vi "test frame felica ask.vi"() -> ()   [LabVIEW 2019]
uses:
  <vilib>/Analysis/3filter.llb/Filter Passband Type.ctl
  <vilib>/addons/Modulation/Analog/support/mod_Set Error Source.vi
  <vilib>/addons/Modulation/Digital/Support/Common/Validators/mod_Generate Filter Coefficients Validate.vi
  <vilib>/addons/Modulation/Digital/General/subVIs/mod_Generate Filter Coefficients.vi
  <vilib>/addons/Modulation/Digital/General/MT Generate ASK system parameters (M).vi
  <vilib>/Waveform/DWDTOps.llb/DWDT Binary U8 to Digital.vi
  <vilib>/addons/Modulation/Analog/MT Modulate AM (DSB).vi
  <vilib>/addons/Modulation/Analog/MT Upconvert Baseband (Real).vi
  <vilib>/express/express analysis/Spectral/Block/exnSpectralBlock spectral measurements RMS poly.vi
  <vilib>/express/express analysis/Spectral/Block/exnSpectralBlock spectral measurements RMS WFM.vi
  <vilib>/Analysis/3filter.llb/Butterworth Filter (DBL).vi
  <vilib>/express/express analysis/Spectral/XNode/ExpressSpectralMeasurementsBlockNode.xnode
  <vilib>/addons/Modulation/niDMT.lvlib
  <vilib>/addons/Modulation/niAMT.lvlib
  <vilib>/Analysis/NI_AALBase.lvlib
panel:
  out "video signal 3":cluster{"t0":dbl, "dt":dbl, "Y":dbl[]}(graph)
  out "video signal 2":cluster{"t0":dbl, "dt":dbl, "Y":dbl[]}(graph)
  in  "command":enum16{"WUP_REQ"}(ring)
  out "error":i32
  out "spectrum analog signal 3":cluster{"t0":dbl, "dt":dbl, "Y":dbl[]}(graph)
  out "Analog signal 2":waveform(dbl)(graph)
  out "spectrum analog signal 2":cluster{"t0":dbl, "dt":dbl, "Y":dbl[]}(graph)
  out "spectrum analog signal":cluster{"t0":dbl, "dt":dbl, "Y":dbl[]}(graph)
  in  "CARRIER (hz)":dbl
  in  "BIT RATE":dbl
  out "LENGHT":u8[](array[numeric]) format="%x"
  out "dt":dbl
  out "Analog signal":waveform(dbl)(graph)
  out "video signal":cluster{"t0":dbl, "dt":dbl, "Y":dbl[]}(graph)
  out "Digital SIGNAL":digitalwaveform(graph)
  out "CRC":u8[](array[numeric]) format="%x"
  in  "Data":u8[](array[numeric]) format="%x"
  in  "SYNC":u8[](array[numeric]) format="%x"
  in  "Preambula":u8[](array[numeric]) format="%x"
  # "0"
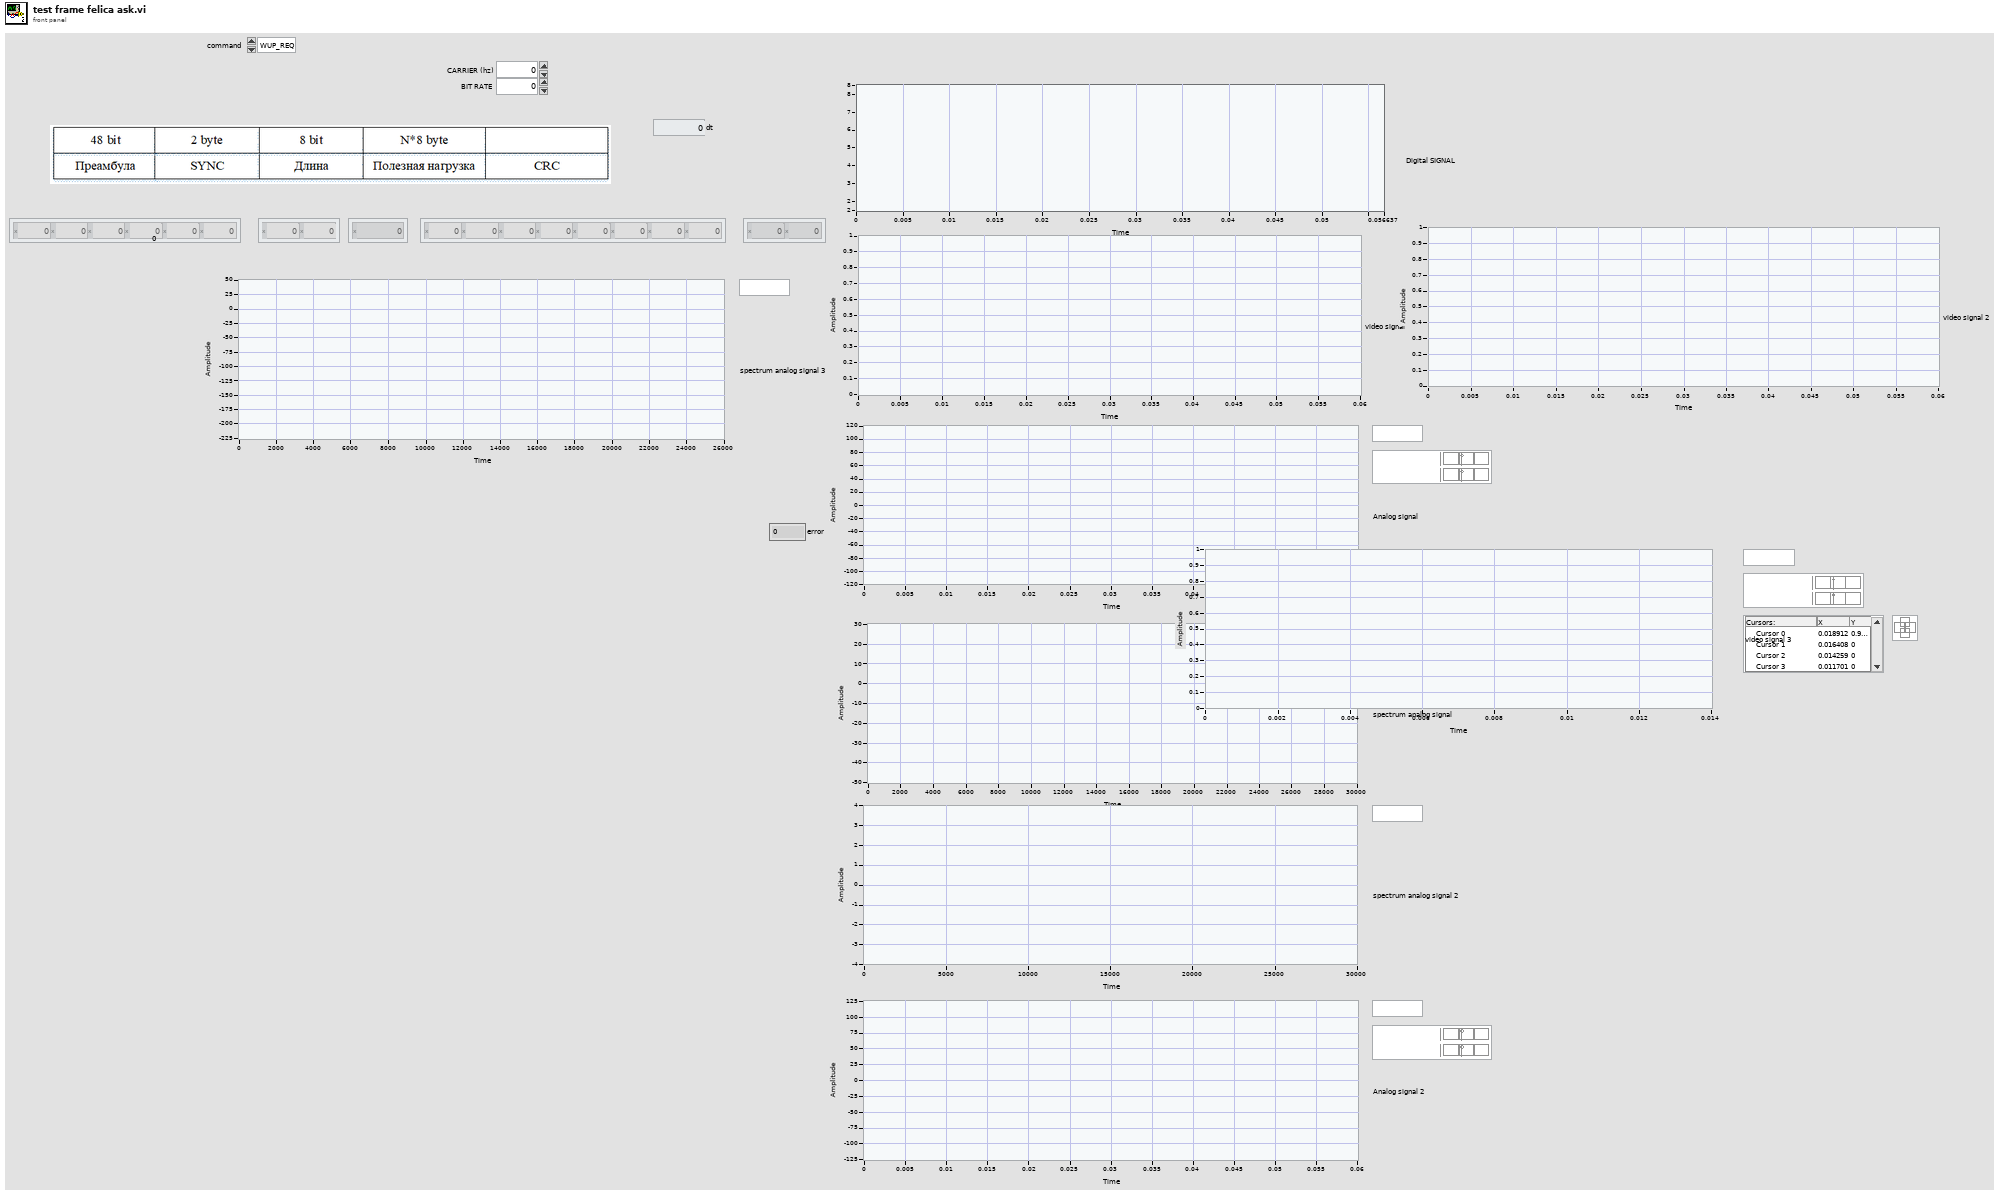
[diagram p1: front panel]
types:
  T1 = enum16{"none", "Raised Cosine", "Root Raised Cos", "Gaussian"}
  T2 = enum16{"FSK", "PSK", "QAM", "MSK", "PAM", "ASK", "CPM"}
  T3 = typedef "NI_AALBase.lvlib/Filter Passband Type.ctl" = enum32{"Lowpass", "Highpass", "Bandpass", "Bandstop"}
  T4 = cluster{"samples per symbol (16)":i32, "symbol map":cdb[]}
  T5 = typedef "niAMT.lvlib/Complex Data Waveform.ctl" = cluster{"t0":dbl, "dt":dbl, "Y":cdb[]}
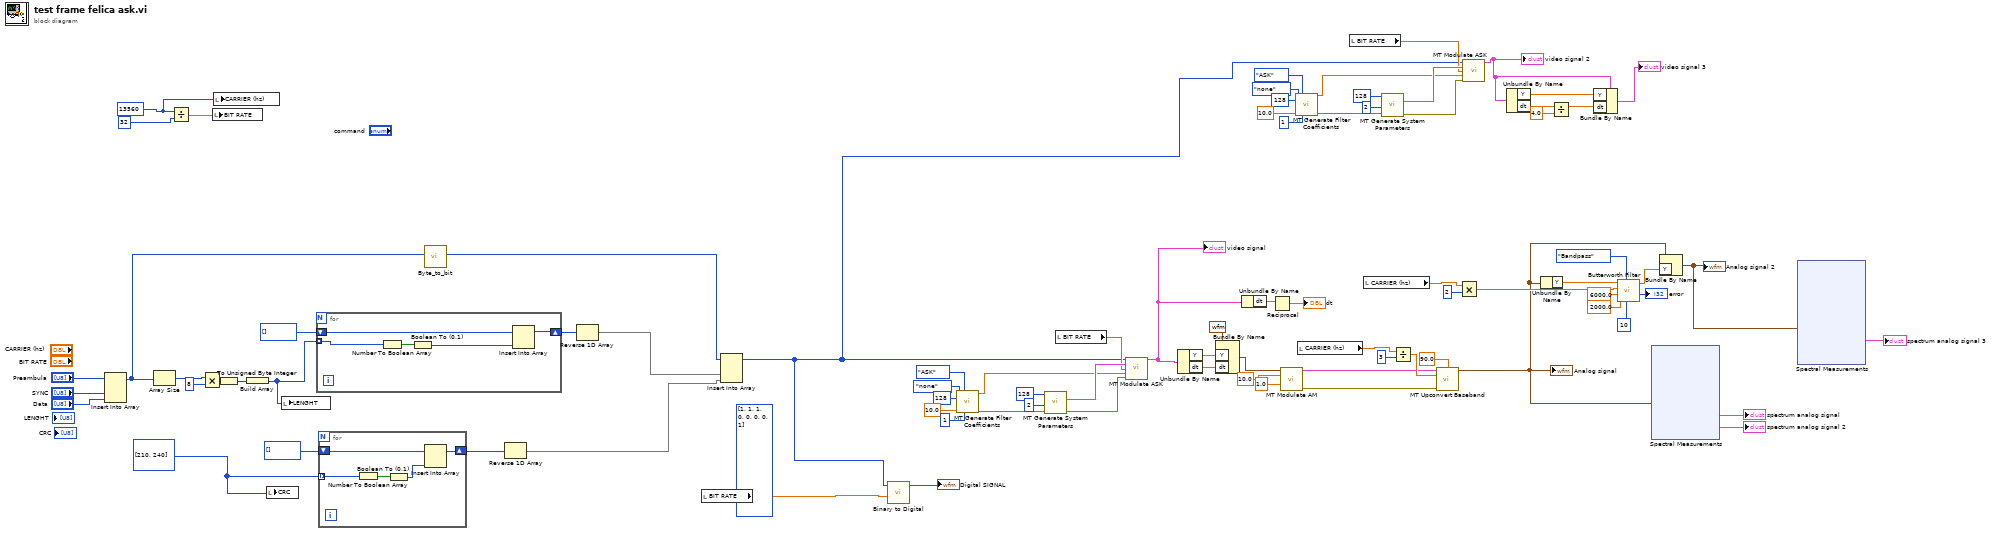
[diagram p0: block diagram]
diagram:
  (unwired) i16[] [1, 1, 1, 0, 0, 0, 0, 1] ("output array")
  w14 = 128 ("pulse shaping samples per symbol (16)")
  w45 = u32 13560
  w61 = 128 ("pulse shaping samples per symbol (16)")
  w48 = u8[] [210, 240] ("CRC")
  n1 = Insert Into Array(array="Preambula", new element #1="SYNC", new element #2="Data") -> (w79:u8[])  [unwired: 1 in]
  n2 = Array Size(array=w79) -> (size(s)=w78:i32)
  n3 = Divide(x=w45, y=u32 32) -> (x/y=w50:dbl)
  n4 = Multiply(x=w78, y=8) -> (x*y=w76:i32)
  n5 = local write "BIT RATE"(w50) -> ()
  n6 = local write "CARRIER (hz)"(w45) -> ()
  n7 = To Unsigned Byte Integer(number=w76) -> (unsigned 8bit integer=w75:u8)
  n8 = Build Array(w75) -> (w47:u8[])
  n9 = local write "CRC"(w48) -> ()
  n10 = local write "LENGHT"(w47) -> ()
  n11 = for {
    tunnel: w47 -> [w87] mode=indexing
    shift-right: [w85] -> w72
    shift-left: i16[] [] -> [w84]
    n12 = Number To Boolean Array(number=w87) -> (Boolean array=w88:bool[])
    n13 = Boolean To (0,1)(Boolean=w88) -> (0, 1=w86:i16[])
    n14 = Insert Into Array(array=w84, new element=w86) -> (w85:i16[])  [unwired: 1 in]
  }
  n15 = for {
    tunnel: w48 -> [w90] mode=indexing
    shift-right: [w92] -> w73
    shift-left: i16[] [] -> [w89]
    n16 = Number To Boolean Array(number=w90) -> (Boolean array=w93:bool[])
    n17 = Boolean To (0,1)(Boolean=w93) -> (0, 1=w91:i16[])
    n18 = Insert Into Array(array=w89, new element=w91) -> (w92:i16[])  [unwired: 1 in]
  }
  n19 = call "Byte_to_bit.vi"("Array of byte"=w79) -> ("Arrray of bit"=w70:u8[])  [unwired: 6 in, 2 out]
  n20 = Reverse 1D Array(array=w73) -> (reversed array=w69:i16[])
  n21 = Reverse 1D Array(array=w72) -> (reversed array=w71:i16[])
  n22 = local read "BIT RATE"() -> (w49:dbl)
  n23 = Insert Into Array(array=w70, new element #1=w71, new element #2=w69) -> (w1:u8[])  [unwired: 1 in]
  n24 = call-poly <vilib>:"Binary to Digital.vi"("sample rate"=w49, "binary array"=w1) -> ("digital waveform"=→"Digital SIGNAL":digitalwaveform)  [unwired: 8 in, 1 out]
  n25 = call <vilib>:"MT Generate Filter Coefficients.vi"("pulse shaping filter (none)"=T1."none", "modulation type"=T2."ASK", "pulse shaping samples per symbol (16)"=w61, "matched samples per symbol (16)"=w61, "filter parameter"=10.0, "filter length (symbols)"=1) -> ("pulse shaping filter coefficients"=w59:dbl[], "error out"=w64:errorcluster)  [unwired: 1 in, 7 out]
  n26 = call-poly <vilib>:"MT Generate System Parameters.vi"("samples per symbol (16)"=128, "M-ASK (2)"=2, "error in (no error)"=w64) -> ("ASK system parameters"=w67:T4, "error out"=w66:errorcluster)  [unwired: 11 out]
  n27 = local read "BIT RATE"() -> (w46:dbl)
  n28 = call <vilib>:"MT Modulate ASK.vi"("input bit stream"=w1, "ASK system parameters"=w67, "symbol rate (Hz)"=w46, "pulse shaping filter coefficients"=w59, "error in (no error)"=w66) -> ("output complex waveform"=w2:T5)  [unwired: 8 in, 2 out]
  "video signal" <- w2
  n29 = Unbundle By Name(w2) -> ("Y"=w41:cdb[], "dt"=w39:dbl)
  n30 = Bundle By Name(cluster=waveform(cdb) {"t0"=timestamp(0 s since 1904-01-01), "dt"=1.0, "Y"=[]} ("waveform"), "Y"=w41, "dt"=w39) -> (w38:waveform(cdb))
  n31 = Unbundle By Name(w2) -> ("dt"=w54:dbl)
  n32 = Reciprocal(x=w54) -> (1/x=→"dt":dbl)
  n33 = call-poly <vilib>:"MT Modulate AM.vi"("message signal"=w38, "modulation index"=10.0, "peak message amplitude"=1.0) -> ("AM modulated waveform"=w37:cluster{"t0":dbl, "dt":dbl, "Y":cdb[]}, "error out"=w43:errorcluster)  [unwired: 11 in]
  n34 = call <vilib>:"MT Generate Filter Coefficients.vi"("pulse shaping filter (none)"=T1."none", "modulation type"=T2."ASK", "pulse shaping samples per symbol (16)"=w14, "matched samples per symbol (16)"=w14, "filter parameter"=10.0, "filter length (symbols)"=1) -> ("pulse shaping filter coefficients"=w12:dbl[], "error out"=w17:errorcluster)  [unwired: 1 in, 7 out]
  n35 = local read "CARRIER (hz)"() -> (w44:dbl)
  n36 = local read "BIT RATE"() -> (w9:dbl)
  n37 = local read "CARRIER (hz)"() -> (w32:dbl)
  n38 = call-poly <vilib>:"MT Generate System Parameters.vi"("samples per symbol (16)"=128, "M-ASK (2)"=2, "error in (no error)"=w17) -> ("ASK system parameters"=w20:T4, "error out"=w19:errorcluster)  [unwired: 11 out]
  n39 = Divide(x=w44, y=u32 3) -> (x/y=w42:dbl)
  n40 = call-poly <vilib>:"MT Upconvert Baseband.vi"("baseband waveform (complex)"=w37, "initial phase (deg)"=90.0, "carrier frequency (Hz)"=w42, "error in (no error)"=w43) -> ("passband waveform"=w26:waveform(dbl))  [unwired: 10 in, 1 out]
  "Analog signal" <- w26
  n41 = Multiply(x=w32, y=u32 2) -> (x*y=w30:dbl)
  n42 = call <vilib>:"MT Modulate ASK.vi"("input bit stream"=w1, "ASK system parameters"=w20, "symbol rate (Hz)"=w9, "pulse shaping filter coefficients"=w12, "error in (no error)"=w19) -> ("output complex waveform"=w3:T5)  [unwired: 8 in, 2 out]
  "video signal 2" <- w3
  n43 = Unbundle By Name(w3) -> ("Y"=w8:cdb[], "dt"=w6:dbl)
  n44 = Unbundle By Name(w26) -> ("Y"=w33:dbl[])
  n45 = Divide(x=w6, y=4.0) -> (x/y=w7:dbl)
  n46 = Bundle By Name(cluster=w3, "Y"=w8, "dt"=w7) -> (→"video signal 3":T5)
  n47 = call-poly <vilib>:"Butterworth Filter.vi"("order"=10, "filter type"=Filter_Passband_Type."Bandpass", "low cutoff freq: fl"=2000.0, "high cutoff freq: fh"=6000.0, "sampling freq: fs"=w30, "X"=w33) -> ("error"=→"error":i32, "Filtered X"=w29:dbl[])  [unwired: 2 in]
  n48 = xnode "Spectral Measurements"("Signals"=w26) -> ("FFT - (RMS)"=→"spectrum analog signal":cluster{"f0":dbl, "df":dbl, "magnitude":dbl[]}, "Phase"=→"spectrum analog signal 2":cluster{"f0":dbl, "df":dbl, "phase":dbl[]})  [unwired: 1 in, 1 out]
  n49 = Bundle By Name(cluster=w26, "Y"=w29) -> (w25:waveform(dbl))
  "Analog signal 2" <- w25
  n50 = xnode "Spectral Measurements"("Signals"=w25) -> ("FFT - (RMS)"=→"spectrum analog signal 3":cluster{"f0":dbl, "df":dbl, "magnitude":dbl[]})  [unwired: 1 in, 2 out]
